vi "INP_READ.vi"(8 "error in (no error)":errorcluster, 11 "Camera Number":u32=1) -> (0 "error out":errorcluster, 1 "INI File Found":bool, 4 "Custom Chip":T1, 5 "ADC and Cleans":T3={"ADC Speed"=-2, "ADC Gain"=-1, "ADC Offset"=-1, "Readout Port"=-1, "Num Cleans"=1, "Num Strips per Clean"=10, "Mini Block Size"=2, "Num Min Blocks"=3, "Continous Cleans"=FALSE, "Skip Serial Reg Clean"=FALSE} {"Readout Port" min=-1 step=1; "ADC Offset" min=-1 step=1; "ADC Gain" min=-1 step=1; "ADC Speed" min=-3 step=1}, 6 "Shutter and Logic Out":T2={"Shutter State"=2, "Open Comp Time "=0, "Close Comp Time"=0, "Logic Out Setting"=1, "Logic Out Invert"=FALSE} {"Logic Out Setting" min=1 max=14 step=1}, 7 "Timing and Temperature":T4={"Exposure"=0.001, "Collection Mode"=1, "Timing Mode"=1, "Trigger Edge"=1, "Temperature"=-10.0} {"Temperature" format="%.2f"; "Trigger Edge" max=7 step=1; "Timing Mode" min=1 max=20 step=1; "Exposure" min=0.0 step=0.001 format="%.3f"})   [LabVIEW 2015]
uses:
  <vilib>/Utility/config.llb/Read Key (String).vi
  <vilib>/Utility/config.llb/Read Key (Double).vi
  <vilib>/Utility/config.llb/Read Key (I32).vi
  <vilib>/Utility/config.llb/Read Key (Boolean).vi
  <vilib>/Utility/config.llb/Read Key (U32).vi
  <vilib>/Utility/config.llb/NI_LVConfig.lvlib
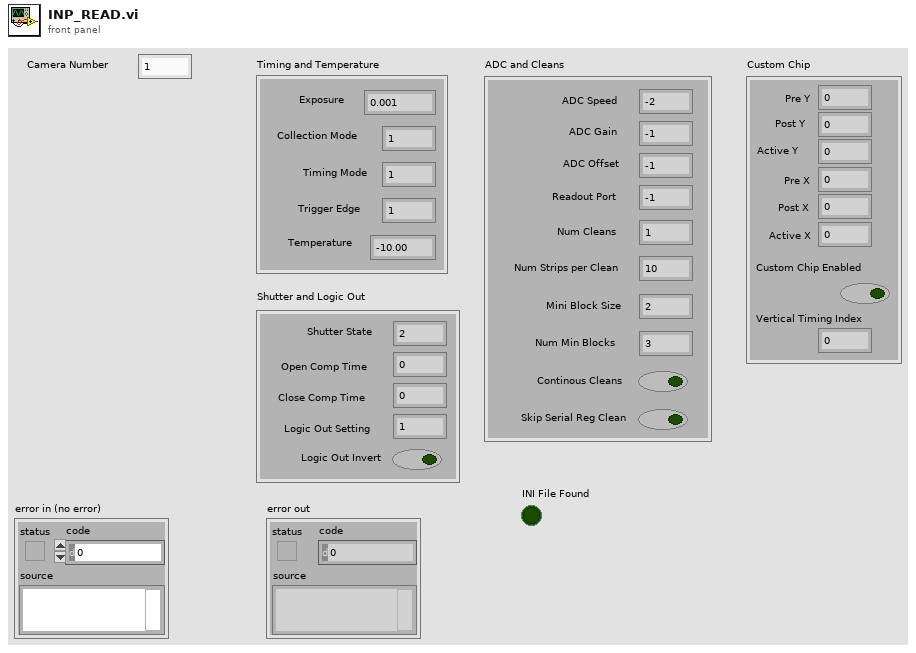
[diagram p1: front panel]
types:
  T1 = cluster{"Pre Y":u32, "Post Y":u32, "Active Y":u32, "Pre X":u32, "Post X":u32, "Active X":u32, "Custom Chip Enabled":bool, "Vertical Timing Index":u32}
  T2 = cluster{"Shutter State":u16, "Open Comp Time ":u32, "Close Comp Time":u32, "Logic Out Setting":u32, "Logic Out Invert":bool}
  T3 = cluster{"ADC Speed":i32, "ADC Gain":i32, "ADC Offset":i32, "Readout Port":i32, "Num Cleans":u32, "Num Strips per Clean":u32, "Mini Block Size":u32, "Num Min Blocks":u32, "Continous Cleans":bool, "Skip Serial Reg Clean":bool}
  T4 = cluster{"Exposure":dbl, "Collection Mode":u32, "Timing Mode":u32, "Trigger Edge":u32, "Temperature":dbl}
  T5 = typedef "NI_LVConfig.lvlib/Config Data RefNum.ctl" = refnum<k1>
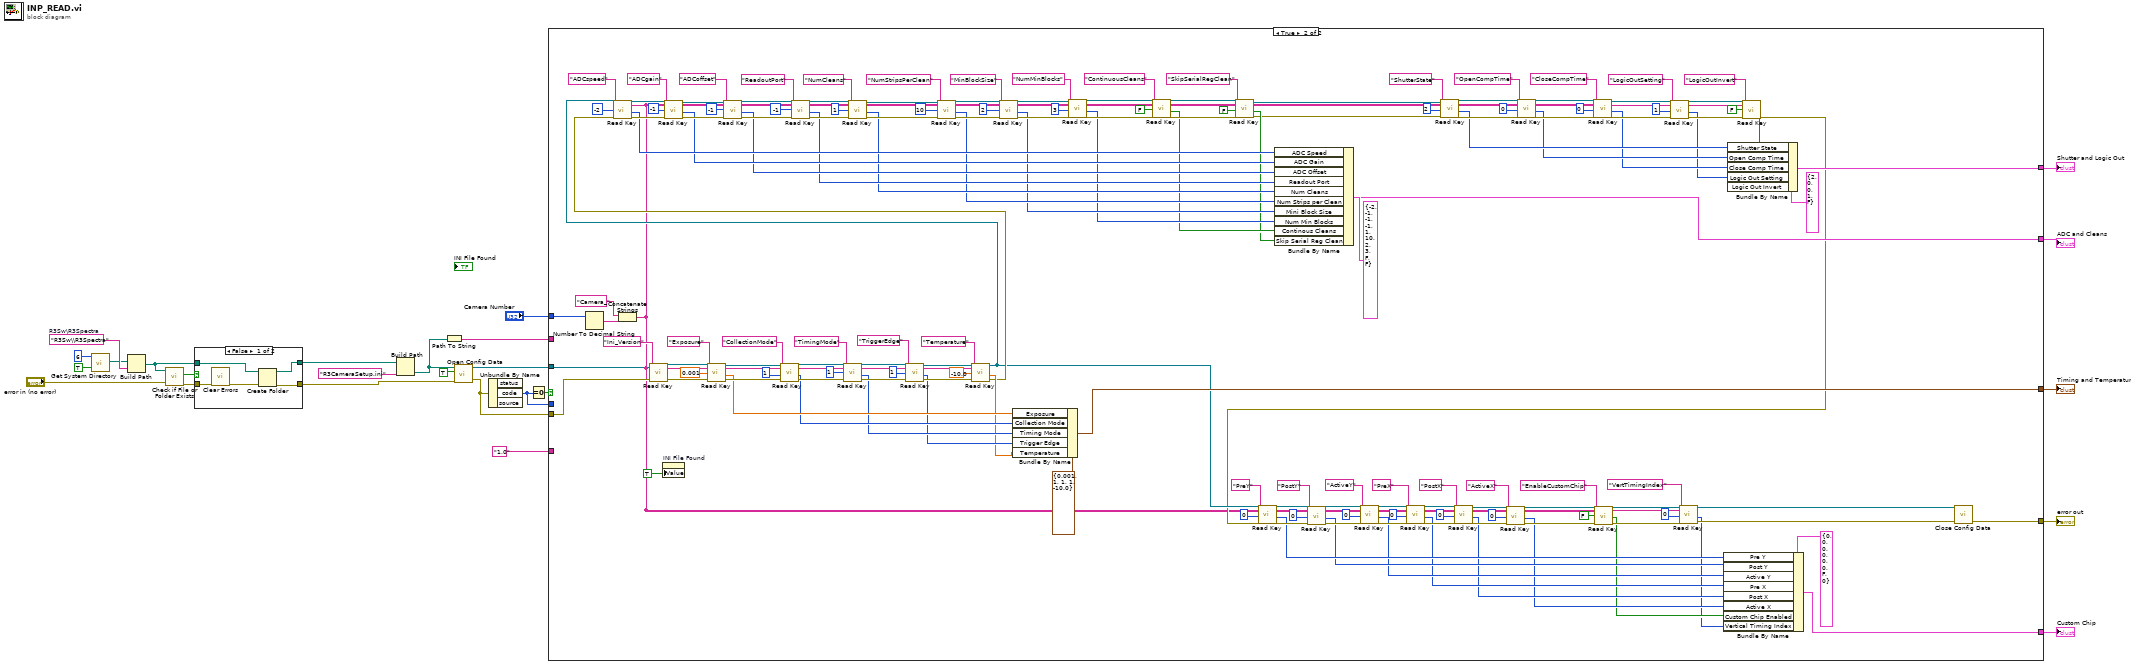
[diagram p0: block diagram]
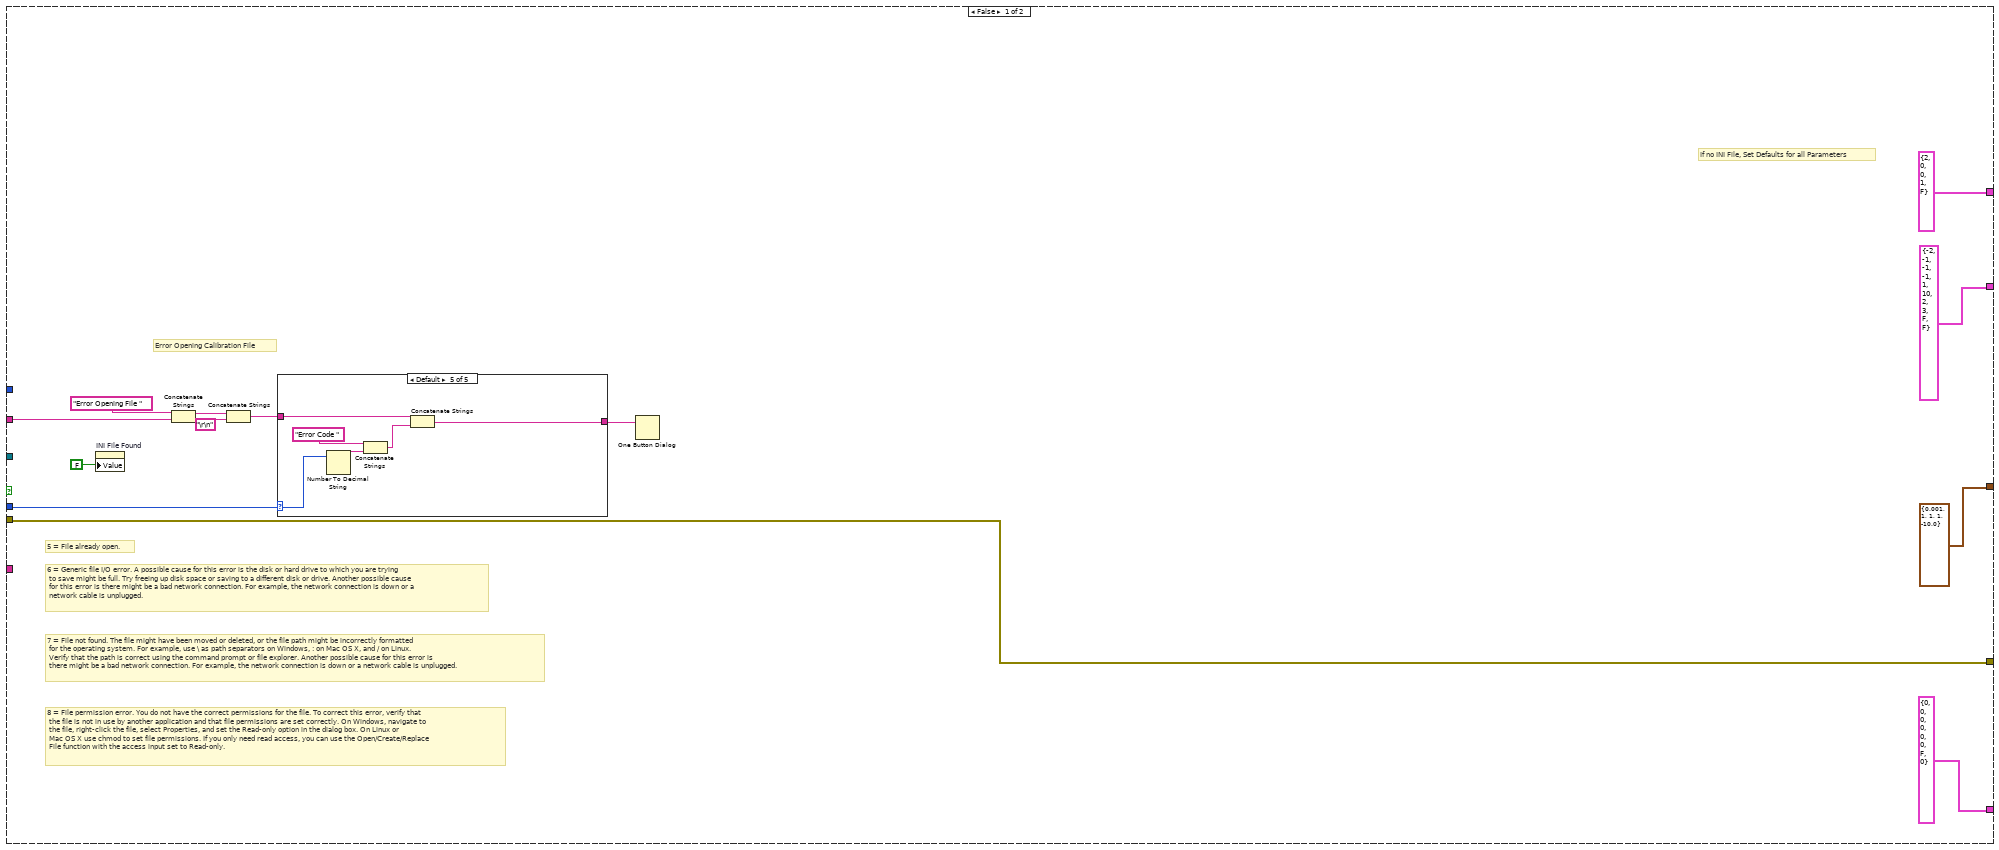
[diagram p3: hidden frame]
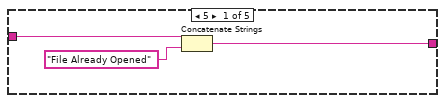
[diagram p4: hidden frame]
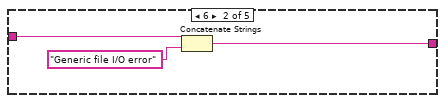
[diagram p5: hidden frame]
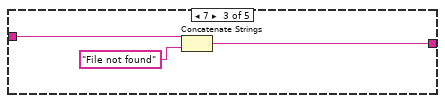
[diagram p6: hidden frame]
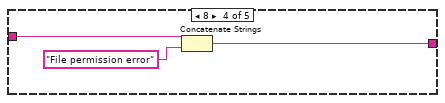
[diagram p7: hidden frame]
diagram:
  w12 = "R3Sw\\R3Spectra"  # R3Sw\R3Spectra
  n1 = call <vilib>:"Get System Directory.vi"("create directory if not found? (F)"=TRUE, "system directory type"=6) -> ("system directory"=w11:path)  [unwired: 9 in]
  n2 = Build Path(base path=w11, name or relative path=w12) -> (appended path=w10:path)
  n3 = call <vilib>:"Check if File or Folder Exists.vi"("error in (no error)"="error in (no error)", "path"=w10) -> ("error out"=w16:errorcluster, "file or folder exists?"=w17:bool)  [unwired: 7 in, 1 out]
  n4 = case shown="False" w17 {
    tunnel: w16 -> [w29 w32]
    tunnel: [w28 w32] -> w15
    tunnel: w10 -> [w30 w31]
    tunnel: [w27 w31] -> w8
    frame False {
      n5 = call <vilib>:"Clear Errors.vi"("error in (no error)"=w29) -> ("error out"=w26:errorcluster)  [unwired: 5 in, 1 out]
      n6 = Create Folder(path (use dialog)=w30, error in=w26) -> (created path=w27:path, error out=w28:errorcluster)  [unwired: 1 in, 1 out]
    }
    frame True {
    }
  }
  n7 = Build Path(base path=w8, name or relative path="R3CameraSetup.ini") -> (appended path=w7:path)
  n8 = Path To String(path=w7) -> (string=w6:string)
  n9 = call <vilib>:"Open Config Data.vi"("error in (no error)"=w15, "create file if necessary (T)"=TRUE, "configuration file path"=w7) -> ("error out"=w22:errorcluster, "refnum"=w23:T5)  [unwired: 6 in, 1 out]
  n10 = Unbundle By Name(w22) -> ("code"=w21:i32)  [unwired: 2 out]
  n11 = Equal To 0?(x=w21) -> (x = 0?=w24:bool)
  n12 = case shown="True" w24 {
    tunnel: w23 -> [_ w218]
    tunnel: w22 -> [w38 w207]
    tunnel: w21 -> [w41 _]
    tunnel: w6 -> [w45 _]
    tunnel: [w38 w200] -> w20
    tunnel: "1.0" -> [_ _]
    tunnel: "Camera Number" -> [_ w181]
    tunnel: [T2 {"Shutter State"=2, "Open Comp Time "=0, "Close Comp Time"=0, "Logic Out Setting"=1, "Logic Out Invert"=FALSE} ("Shutter and Logic Out") w113] -> w4
    tunnel: [T3 {"ADC Speed"=-2, "ADC Gain"=-1, "ADC Offset"=-1, "Readout Port"=-1, "Num Cleans"=1, "Num Strips per Clean"=10, "Mini Block Size"=2, "Num Min Blocks"=3, "Continous Cleans"=FALSE, "Skip Serial Reg Clean"=FALSE} ("ADC and Cleans") w112] -> w3
    tunnel: [T4 {"Exposure"=0.001, "Collection Mode"=1, "Timing Mode"=1, "Trigger Edge"=1, "Temperature"=-10.0} ("Timing and Temperature") w111] -> w2
    tunnel: [T1 {"Pre Y"=0, "Post Y"=0, "Active Y"=0, "Pre X"=0, "Post X"=0, "Active X"=0, "Custom Chip Enabled"=FALSE, "Vertical Timing Index"=0} ("Custom Chip") w64] -> w1
    frame False {
      # "If no INI File, Set Defaults for all Parameters"
      # "8 = File permission error. You do not have the correct permissions for the file. To correct this error, verify that\n the file is not in use by another application and that file permissions are set correctly. On Windows, navigate to\n the file, right-click the file, select Properties, and set the Read-only option in the dialog box. On Linux or\n Mac OS X use chmod to set file permissions. If you only need read access, you can use the Open/Create/Replace\n File function with the access input set to Read-only."
      # "7 = File not found. The file might have been moved or deleted, or the file path might be incorrectly formatted\n for the operating system. For example, use \\ as path separators on Windows, : on Mac OS X, and / on Linux.\n Verify that the path is correct using the command prompt or file explorer. Another possible cause for this error is\n there might be a bad network connection. For example, the network connection is down or a network cable is unplugged."
      # "6 = Generic file I/O error. A possible cause for this error is the disk or hard drive to which you are trying\n to save might be full. Try freeing up disk space or saving to a different disk or drive. Another possible cause\n for this error is there might be a bad network connection. For example, the network connection is down or a\n network cable is unplugged."
      # "5 = File already open."
      # "Error Opening Calibration File"
      n13 = property on="INI File Found" class="Bool (strict)"("Value"=FALSE) -> ()  [unwired: 2 in, 2 out]
      n14 = Concatenate Strings("Error Opening File ", w45) -> (w42:string)
      n15 = Concatenate Strings(w42, "\r\n") -> (w40:string)
      n16 = case shown="Default" w41 {
        selector: w41 -> [_ _ _ _ w61]
        tunnel: w40 -> [w47 w50 w53 w56 w63]
        tunnel: [w46 w49 w52 w55 w62] -> w39
        frame 5 {
          n17 = Concatenate Strings(w47, "File Already Opened") -> (w46:string)
        }
        frame 6 {
          n18 = Concatenate Strings(w50, "Generic file I/O error") -> (w49:string)
        }
        frame 7 {
          n19 = Concatenate Strings(w53, "File not found") -> (w52:string)
        }
        frame 8 {
          n20 = Concatenate Strings(w56, "File permission error") -> (w55:string)
        }
        frame Default {
          n21 = Number To Decimal String(number=w61) -> (decimal integer string=w60:string)  [unwired: 1 in]
          n22 = Concatenate Strings("Error Code ", w60) -> (w58:string)
          n23 = Concatenate Strings(w63, w58) -> (w62:string)
        }
      }
      n24 = One Button Dialog(message=w39) -> ()  [unwired: 1 in, 1 out]
    }
    frame True {
      n25 = Number To Decimal String(number=w181) -> (decimal integer string=w182:string)  [unwired: 1 in]
      n26 = Concatenate Strings("Camera_", w182) -> (w76:string)
      n27 = call-poly <vilib>:"Read Key.vi"("section"=w76, "error in (no error)"=w207, "key"="Ini_Version", "refnum"=w218) -> ("error out"=w206:errorcluster, "refnum out"=w216:T5)  [unwired: 4 in, 2 out]
      n28 = property on="INI File Found" class="Bool (strict)"("Value"=TRUE) -> ()  [unwired: 2 in, 2 out]
      n29 = call-poly <vilib>:"Read Key.vi"("section"=w76, "error in (no error)"=w206, "default value"=0.001 ("Exposure"), "key"="Exposure", "refnum"=w216) -> ("error out"=w201:errorcluster, "value"=w174:dbl, "refnum out"=w215:T5)  [unwired: 3 in, 1 out]
      n30 = call-poly <vilib>:"Read Key.vi"("section"=w76, "error in (no error)"=w201, "default value"=1, "key"="CollectionMode", "refnum"=w215) -> ("error out"=w205:errorcluster, "value"=w173:i32, "refnum out"=w214:T5)  [unwired: 3 in, 1 out]
      n31 = call-poly <vilib>:"Read Key.vi"("section"=w76, "error in (no error)"=w205, "default value"=u32 1 ("Timing Mode"), "key"="TimingMode", "refnum"=w214) -> ("error out"=w204:errorcluster, "value"=w172:i32, "refnum out"=w212:T5)  [unwired: 3 in, 1 out]
      n32 = call-poly <vilib>:"Read Key.vi"("section"=w76, "error in (no error)"=w204, "default value"=u32 1 ("Trigger Edge"), "key"="TriggerEdge", "refnum"=w212) -> ("error out"=w203:errorcluster, "value"=w171:i32, "refnum out"=w211:T5)  [unwired: 3 in, 1 out]
      n33 = call-poly <vilib>:"Read Key.vi"("section"=w76, "error in (no error)"=w203, "default value"=-10.0 ("Temperature"), "key"="Temperature", "refnum"=w211) -> ("error out"=w109:errorcluster, "value"=w170:dbl, "refnum out"=w86:T5)  [unwired: 3 in, 1 out]
      n34 = call-poly <vilib>:"Read Key.vi"("section"=w76, "error in (no error)"=w109, "default value"=-2 ("ADC Speed"), "key"="ADCspeed", "refnum"=w86) -> ("error out"=w202:errorcluster, "value"=w149:i32, "refnum out"=w208:T5)  [unwired: 3 in, 1 out]
      n35 = call-poly <vilib>:"Read Key.vi"("section"=w76, "error in (no error)"=w202, "default value"=-1 ("ADC Gain"), "key"="ADCgain", "refnum"=w208) -> ("error out"=w194:errorcluster, "value"=w148:i32, "refnum out"=w189:T5)  [unwired: 3 in, 1 out]
      n36 = call-poly <vilib>:"Read Key.vi"("section"=w76, "error in (no error)"=w194, "default value"=-1 ("ADC Offset"), "key"="ADCoffset", "refnum"=w189) -> ("error out"=w193:errorcluster, "value"=w147:i32, "refnum out"=w188:T5)  [unwired: 3 in, 1 out]
      n37 = call-poly <vilib>:"Read Key.vi"("section"=w76, "error in (no error)"=w193, "default value"=-1 ("Readout Port"), "key"="ReadoutPort", "refnum"=w188) -> ("error out"=w192:errorcluster, "value"=w146:i32, "refnum out"=w187:T5)  [unwired: 3 in, 1 out]
      n38 = call-poly <vilib>:"Read Key.vi"("section"=w76, "error in (no error)"=w192, "default value"=u32 1 ("Num Cleans"), "key"="NumCleans", "refnum"=w187) -> ("error out"=w191:errorcluster, "value"=w145:i32, "refnum out"=w186:T5)  [unwired: 3 in, 1 out]
      n39 = call-poly <vilib>:"Read Key.vi"("section"=w76, "error in (no error)"=w191, "default value"=u32 10 ("Num Strips per Clean"), "key"="NumStripsPerClean", "refnum"=w186) -> ("error out"=w190:errorcluster, "value"=w144:i32, "refnum out"=w185:T5)  [unwired: 3 in, 1 out]
      n40 = call-poly <vilib>:"Read Key.vi"("section"=w76, "error in (no error)"=w190, "default value"=u32 2 ("Mini Block Size"), "key"="MinBlockSize", "refnum"=w185) -> ("error out"=w156:errorcluster, "value"=w143:i32, "refnum out"=w159:T5)  [unwired: 3 in, 1 out]
      n41 = Bundle By Name(cluster=T4 {"Exposure"=0.001, "Collection Mode"=1, "Timing Mode"=1, "Trigger Edge"=1, "Temperature"=-10.0} ("Timing and Temperature"), "Exposure"=w174, "Collection Mode"=w173, "Timing Mode"=w172, "Trigger Edge"=w171, "Temperature"=w170) -> (w111:T4)
      n42 = call-poly <vilib>:"Read Key.vi"("section"=w76, "error in (no error)"=w156, "default value"=u32 3 ("Num Min Blocks"), "key"="NumMinBlocks", "refnum"=w159) -> ("error out"=w155:errorcluster, "value"=w142:i32, "refnum out"=w158:T5)  [unwired: 3 in, 1 out]
      n43 = call-poly <vilib>:"Read Key.vi"("section"=w76, "error in (no error)"=w155, "default value"=FALSE ("Continous Cleans"), "key"="ContinuousCleans", "refnum"=w158) -> ("error out"=w154:errorcluster, "value"=w141:bool, "refnum out"=w157:T5)  [unwired: 3 in, 1 out]
      n44 = call-poly <vilib>:"Read Key.vi"("section"=w76, "error in (no error)"=w154, "default value"=FALSE ("Continous Cleans"), "key"="SkipSerialRegClean", "refnum"=w157) -> ("error out"=w138:errorcluster, "value"=w140:bool, "refnum out"=w137:T5)  [unwired: 3 in, 1 out]
      n45 = Bundle By Name(cluster=T3 {"ADC Speed"=-2, "ADC Gain"=-1, "ADC Offset"=-1, "Readout Port"=-1, "Num Cleans"=1, "Num Strips per Clean"=10, "Mini Block Size"=2, "Num Min Blocks"=3, "Continous Cleans"=FALSE, "Skip Serial Reg Clean"=FALSE} ("ADC and Cleans"), "ADC Speed"=w149, "ADC Gain"=w148, "ADC Offset"=w147, "Readout Port"=w146, "Num Cleans"=w145, "Num Strips per Clean"=w144, "Mini Block Size"=w143, "Num Min Blocks"=w142, "Continous Cleans"=w141, "Skip Serial Reg Clean"=w140) -> (w112:T3)
      n46 = call-poly <vilib>:"Read Key.vi"("section"=w76, "error in (no error)"=w138, "default value"=u16 2 ("Shutter State"), "key"="ShutterState", "refnum"=w137) -> ("error out"=w121:errorcluster, "value"=w118:i32, "refnum out"=w128:T5)  [unwired: 3 in, 1 out]
      n47 = call-poly <vilib>:"Read Key.vi"("section"=w76, "error in (no error)"=w121, "default value"=u16 0 ("Shutter State"), "key"="OpenCompTime", "refnum"=w128) -> ("error out"=w122:errorcluster, "value"=w117:i32, "refnum out"=w127:T5)  [unwired: 3 in, 1 out]
      n48 = call-poly <vilib>:"Read Key.vi"("section"=w76, "error in (no error)"=w122, "default value"=u16 0 ("Shutter State"), "key"="CloseCompTime", "refnum"=w127) -> ("error out"=w123:errorcluster, "value"=w116:i32, "refnum out"=w126:T5)  [unwired: 3 in, 1 out]
      n49 = call-poly <vilib>:"Read Key.vi"("section"=w76, "error in (no error)"=w123, "default value"=u16 1 ("Shutter State"), "key"="LogicOutSetting", "refnum"=w126) -> ("error out"=w124:errorcluster, "value"=w115:i32, "refnum out"=w125:T5)  [unwired: 3 in, 1 out]
      n50 = call-poly <vilib>:"Read Key.vi"("section"=w76, "error in (no error)"=w124, "default value"=FALSE ("Continous Cleans"), "key"="LogicOutInvert", "refnum"=w125) -> ("error out"=w83:errorcluster, "value"=w114:bool)  [unwired: 3 in, 2 out]
      n51 = call-poly <vilib>:"Read Key.vi"("section"=w76, "error in (no error)"=w83, "default value"=u16 0 ("Shutter State"), "key"="PreY", "refnum"=w86) -> ("error out"=w82:errorcluster, "value"=w72:u32, "refnum out"=w85:T5)  [unwired: 3 in, 1 out]
      n52 = call-poly <vilib>:"Read Key.vi"("section"=w76, "error in (no error)"=w82, "default value"=u16 0 ("Shutter State"), "key"="PostY", "refnum"=w85) -> ("error out"=w81:errorcluster, "value"=w71:u32, "refnum out"=w84:T5)  [unwired: 3 in, 1 out]
      n53 = call-poly <vilib>:"Read Key.vi"("section"=w76, "error in (no error)"=w81, "default value"=u16 0 ("Shutter State"), "key"="ActiveY", "refnum"=w84) -> ("error out"=w92:errorcluster, "value"=w70:u32, "refnum out"=w99:T5)  [unwired: 3 in, 1 out]
      n54 = call-poly <vilib>:"Read Key.vi"("section"=w76, "error in (no error)"=w92, "default value"=u16 0 ("Shutter State"), "key"="PreX", "refnum"=w99) -> ("error out"=w93:errorcluster, "value"=w69:u32, "refnum out"=w98:T5)  [unwired: 3 in, 1 out]
      n55 = call-poly <vilib>:"Read Key.vi"("section"=w76, "error in (no error)"=w93, "default value"=u16 0 ("Shutter State"), "key"="PostX", "refnum"=w98) -> ("error out"=w94:errorcluster, "value"=w68:u32, "refnum out"=w97:T5)  [unwired: 3 in, 1 out]
      n56 = call-poly <vilib>:"Read Key.vi"("section"=w76, "error in (no error)"=w94, "default value"=u16 0 ("Shutter State"), "key"="ActiveX", "refnum"=w97) -> ("error out"=w95:errorcluster, "value"=w67:u32, "refnum out"=w96:T5)  [unwired: 3 in, 1 out]
      n57 = call-poly <vilib>:"Read Key.vi"("section"=w76, "error in (no error)"=w95, "default value"=FALSE ("Continous Cleans"), "key"="EnableCustomChip", "refnum"=w96) -> ("error out"=w77:errorcluster, "value"=w66:bool, "refnum out"=w78:T5)  [unwired: 3 in, 1 out]
      n58 = call-poly <vilib>:"Read Key.vi"("section"=w76, "error in (no error)"=w77, "default value"=u16 0 ("Shutter State"), "key"="VertTimingIndex", "refnum"=w78) -> ("error out"=w75:errorcluster, "value"=w65:u32, "refnum out"=w74:T5)  [unwired: 3 in, 1 out]
      n59 = Bundle By Name(cluster=T1 {"Pre Y"=0, "Post Y"=0, "Active Y"=0, "Pre X"=0, "Post X"=0, "Active X"=0, "Custom Chip Enabled"=FALSE, "Vertical Timing Index"=0} ("Custom Chip"), "Pre Y"=w72, "Post Y"=w71, "Active Y"=w70, "Pre X"=w69, "Post X"=w68, "Active X"=w67, "Custom Chip Enabled"=w66, "Vertical Timing Index"=w65) -> (w64:T1)
      n60 = Bundle By Name(cluster=T2 {"Shutter State"=2, "Open Comp Time "=0, "Close Comp Time"=0, "Logic Out Setting"=1, "Logic Out Invert"=FALSE} ("Shutter and Logic Out"), "Shutter State"=w118, "Open Comp Time"=w117, "Close Comp Time"=w116, "Logic Out Setting"=w115, "Logic Out Invert"=w114) -> (w113:T2)
      n61 = call <vilib>:"Close Config Data.vi"("error in (no error)"=w75, "refnum"=w74) -> ("error out"=w200:errorcluster)  [unwired: 8 in, 1 out]
    }
  }
  "error out" <- w20
  "Timing and Temperature" <- w2
  "ADC and Cleans" <- w3
  "Shutter and Logic Out" <- w4
  "Custom Chip" <- w1
